vi "Send command ADC.vi"(8 "error in (no error)":errorcluster, 9 "Canal":string(combo), 10 "Marca":string, 11 "object in":refnum<class "Arduino.lvclass">) -> (0 "error out":errorcluster, 1 "Expected response":string, 2 "Command":string, 3 "object out":refnum<class "Arduino.lvclass">)   [LabVIEW 2020, in "Arduino.lvclass"]
uses:
  Arduino.lvclass
  Arduino.lvclass/Arduino.ctl
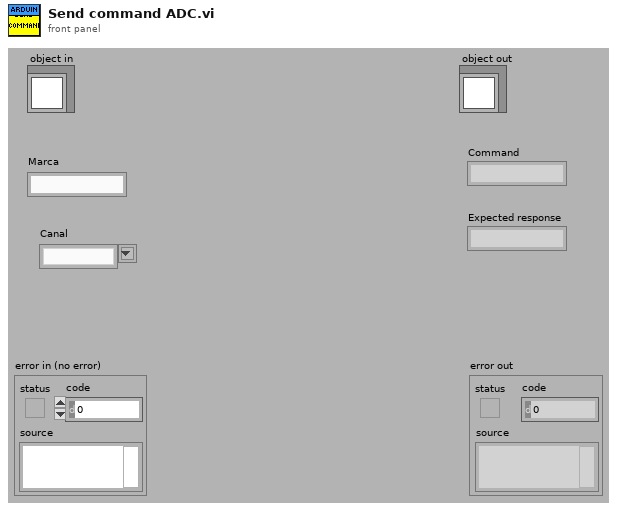
[diagram p1: front panel]
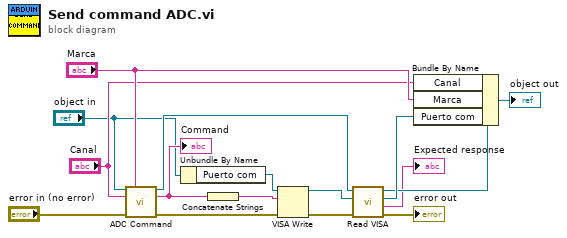
[diagram p0: block diagram]
diagram:
  n1 = call-dynamic "ADC Command.vi"("object in"="object in", "Marca"="Marca", "Canal"="Canal", "error in (no error)"="error in (no error)") -> ("object out"=w12:refnum<class "Arduino.lvclass">, "Command"=w5:string, "error out"=w15:errorcluster)  [unwired: 8 in, 1 out]
  "Command" <- w5
  n2 = Unbundle By Name("object in") -> ("Puerto com"=w1:refnum<visa-resource-name>)
  n3 = Concatenate Strings(w5) -> (w16:string)
  n4 = VISA Write(VISA resource name=w1, write buffer=w16, error in (no error)=w15) -> (VISA resource name out=w14:refnum<visa-resource-name>, error out=w13:errorcluster)  [unwired: 1 out]
  n5 = call-dynamic "Read VISA.vi"("error in (no error)"=w13, "VISA Refnum in"=w14, "Serial Device in"=w12) -> ("error out"=→"error out":errorcluster, "Serial Response"=→"Expected response":string, "VISA resource name out"=w11:refnum<visa-resource-name>, "Serial Device out"=w10:refnum<class "Arduino.lvclass">)  [unwired: 5 in]
  n6 = Bundle By Name(cluster=w10, "Canal"="Canal", "Marca"="Marca", "Puerto com"=w11) -> (→"object out":refnum<class "Arduino.lvclass">)
